vi "Reset - NI.vi"(8 "error in (no error)":errorcluster, 11 "instrument handle":refnum<k15>) -> (0 "error out":errorcluster, 3 "instrument handle out":refnum<k15>)   [LabVIEW 2020]
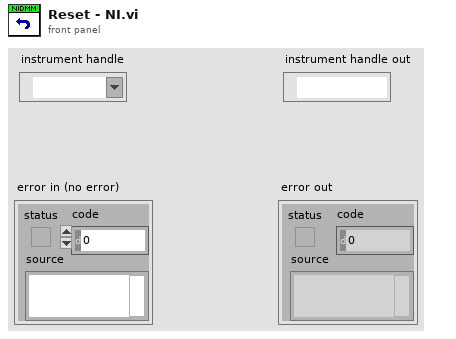
[diagram p1: front panel]
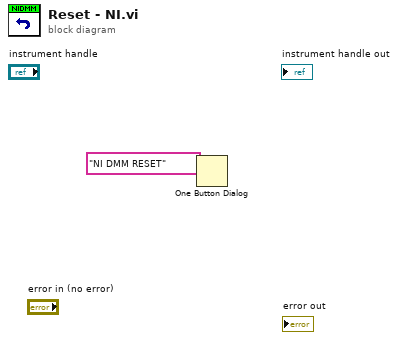
[diagram p0: block diagram]
diagram:
  n1 = One Button Dialog(message="NI DMM RESET") -> ()  [unwired: 1 in, 1 out]
